vi "Pcre2SubstringFromSubjectByNumber8 (bsa).vi"(8 "error in":errorcluster, 9 "Number":i32, 10 "Subject":string, 11 "pMatchData":u64 format="%.0x") -> (0 "error out":errorcluster, 2 "Substring":string, 3 "pMatchData":u64 format="%.0x", 4 "AfterSubstring":string, 5 "BeforeSubstring":string)   [LabVIEW 2021, in "libpcre2-8.lvlib"]
uses:
  libpcre2-8.lvlib
  Pcre2GetOvectorPointer8.vi
  Pcre2MoOfSubstrNumFmOv.vi
  Pcre2ErrorNull.vi
  Pcre2LibError.vi
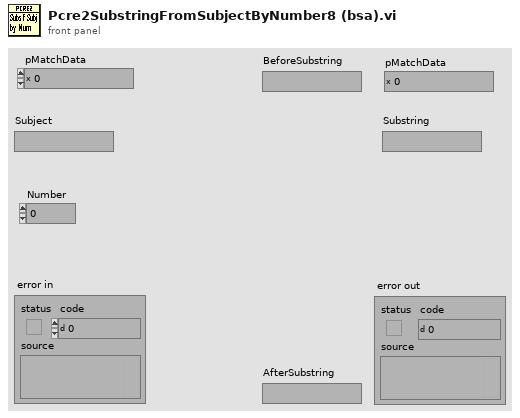
[diagram p1: front panel]
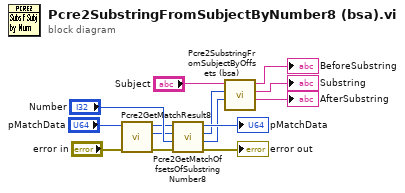
[diagram p0: block diagram]
diagram:
  n1 = call "Pcre2GetMatchResult8.vi"("error in"="error in", "pMatchData"="pMatchData") -> ("error out"=w8:errorcluster, "MatchResult"=w7:i32, "pMatchData"=w9:u64)  [unwired: 7 in]
  n2 = call "Pcre2GetMatchOffsetsOfSubstringNumber8.vi"("error in"=w8, "Number"="Number", "MatchResult"=w7, "pMatchData"=w9) -> ("error out"=→"error out":errorcluster, "OffsetPastMatch"=w1:i32, "MatchOffset"=w2:i32, "pMatchData"=→"pMatchData":u64)  [unwired: 4 in]
  n3 = call "Pcre2SubstringFromSubjectByOffsets (bsa).vi"("OffsetPastMatch"=w1, "MatchOffset"=w2, "Subject"="Subject") -> ("AfterSubstring"=→"AfterSubstring":string, "Substring"=→"Substring":string, "BeforeSubstring"=→"BeforeSubstring":string)  [unwired: 6 in]
